vi "JoystickToBool (SubVI).vi"(10 "Threshold":dbl, 11 "Axis":dbl) -> (2 "AutoForward":bool, 3 "AutoTurn":bool)   [LabVIEW 2018, in "Joysticks.lvlib" / "Two Drivers.lvclass"]
doc: "This VI is currently unused in code but its orginal intent was to use the forward backward direction on a joystick to implement vison control."
uses:
  Two Drivers.lvclass
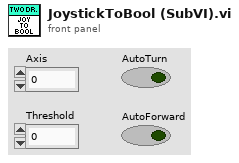
[diagram p1: front panel]
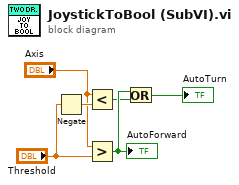
[diagram p0: block diagram]
diagram:
  n1 = Negate(x="Threshold") -> (-x=w2:dbl)
  n2 = Less?(x="Axis", y=w2) -> (x < y?=w4:bool)
  n3 = Greater?(x="Axis", y="Threshold") -> (0:w6:bool)
  "AutoForward" <- w6
  n4 = Or(x=w6, y=w4) -> (x .or. y?=→"AutoTurn":bool)
